vi "reheat.vi"(8 "error in (no error)":errorcluster, 11 "Stove in":refnum<class "Stove.lvclass">) -> (0 "error out":errorcluster, 3 "Stove out":refnum<class "Stove.lvclass">)   [LabVIEW 2011, in "Stove.lvclass"]
uses:
  Stove.lvclass
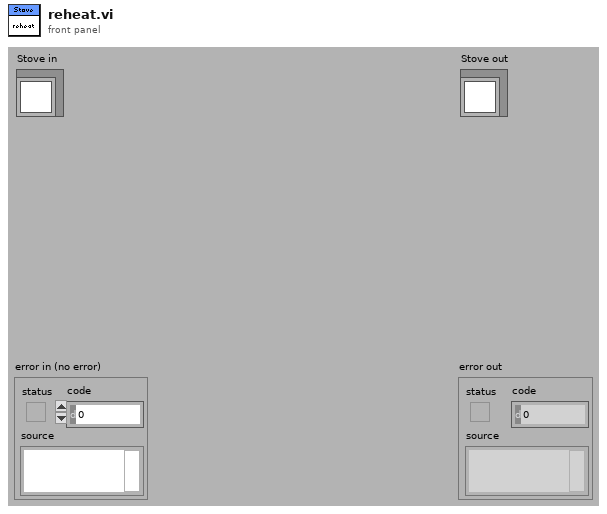
[diagram p1: front panel]
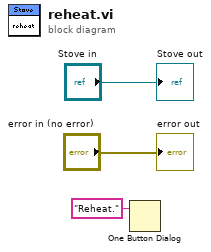
[diagram p0: block diagram]
diagram:
  n1 = One Button Dialog(message="Reheat.") -> ()  [unwired: 1 in, 1 out]
  "error out" <- "error in (no error)"
  "Stove out" <- "Stove in"
